vi "test FPGA.vi"() -> ()   [LabVIEW 2017]
uses:
  <vilib>/LabVIEW Targets/FPGA/cRIO/shared/nicrio_ModuleControls/nicrio_cRIO-9775_TriggerSlope.ctl
  <vilib>/LabVIEW Targets/FPGA/cRIO/shared/nicrio_ModuleControls/nicrio_BasicConversionTime.ctl
  <vilib>/LabVIEW Targets/FPGA/cRIO/shared/nicrio_ModuleControls/nicrio_cRIO-9775_RecordDataRates4ChansRing.ctl
  <vilib>/rvi/Emulation/niFpgaGetClockAttributes.vi
  <vilib>/rvi/Emulation/niFpgaSctlEmulationGetInTimedLoop.vi
  <vilib>/rvi/Emulation/niFpgaEmulationReportErrorSimple.vi
  <vilib>/rvi/eio/common/nirviEmuTemplateMethod_errors.vi
  <vilib>/rvi/Emulation/niFpgaCriticalErrorInLSC.vi
  <vilib>/rvi/eio/common/nirviEmuTemplatePropertySet_errors.vi
  <vilib>/rvi/interface/RandomDataEmulation/niFpgaRandomDataHandleErrors.vi
  <vilib>/eio/EIOMethodNode/EIOMethodNode.xnode
  <vilib>/eio/EIONode/EIONode.xnode
  <vilib>/eio/EIOPropertyNode/EIOPropertyNode.xnode
  <vilib>/rvi/DataTransferAndStorage/Container/XNode/niFpgaContainer.xnode
  <vilib>/rvi/interface/RandomDataEmulation/nirviRandomDataFpgaReadWriteTemplate.vi
  <vilib>/rvi/eio/common/nirviEmuTemplatePropertyGet_errors.vi
  <vilib>/rvi/eio/common/nirviEmuTemplatePropertyGet_noerrors.vi
  <vilib>/rvi/eio/common/nirviEmuTemplatePropertySet_noerrors.vi
panel:
  in  "stop":bool
  in  "Timeout":i32
  in  "Record Samples":u32=25
  in  "Record PreTrigger Samples":u32=1
  in  "Record Data Rate":T1=1 items=["20.000 MS/s (NI 9775)"=1, "10.00 MS/s (NI 9775)"=2, "6.667 MS/s (NI 9775)"=3, "5.000 MS/s (NI 9775)"=4, "2.500 MS/s (NI 9775)"=8, "1.667 MS/s (NI 9775)"=12, "1.250 MS/s (NI 9775)"=16, "1.000 MS/s (NI 9775)"=20, "833.333 KS/s (NI 9775)"=24, "714.286 KS/s (NI 9775)"=28, "625.000 KS/s (NI 9775)"=32, "555.556 KS/s (NI 9775)"=36, "500.000 KS/s (NI 9775)"=40, "454.545 KS/s (NI 9775)"=44, "416.667 KS/s (NI 9775)"=48, "384.615 KS/s (NI 9775)"=52, "357.143 KS/s (NI 9775)"=56, "333.333 KS/s (NI 9775)"=60, "312.500 KS/s (NI 9775)"=64, "294.118 KS/s (NI 9775)"=68, "277.778 KS/s (NI 9775)"=72, "263.158 KS/s (NI 9775)"=76, "250.000 KS/s (NI 9775)"=80, "238.095 KS/s (NI 9775)"=84, "227.273 KS/s (NI 9775)"=88, "217.391 KS/s (NI 9775)"=92, "208.333 KS/s (NI 9775)"=96, "200.000 KS/s (NI 9775)"=100, "192.308 KS/s (NI 9775)"=104, "185.185 KS/s (NI 9775)"=108, "178.571 KS/s (NI 9775)"=112, "172.414 KS/s (NI 9775)"=116, "166.667 KS/s (NI 9775)"=120, "161.290 KS/s (NI 9775)"=124, "156.250 KS/s (NI 9775)"=128, "151.515 KS/s (NI 9775)"=132, "147.059 KS/s (NI 9775)"=136, "142.857 KS/s (NI 9775)"=140, "138.889 KS/s (NI 9775)"=144, "135.135 KS/s (NI 9775)"=148, "131.579 KS/s (NI 9775)"=152, "128.205 KS/s (NI 9775)"=156, "125.000 KS/s (NI 9775)"=160, "121.951 KS/s (NI 9775)"=164, "119.048 KS/s (NI 9775)"=168, "116.279 KS/s (NI 9775)"=172, "113.636 KS/s (NI 9775)"=176, "111.111 KS/s (NI 9775)"=180, "108.696 KS/s (NI 9775)"=184, "106.383 KS/s (NI 9775)"=188, "104.167 KS/s (NI 9775)"=192, "102.041 KS/s (NI 9775)"=196, "100.000 KS/s (NI 9775)"=200, "50.000 KS/s (NI 9775)"=400, "33.333 KS/s (NI 9775)"=600, "25.000 KS/s (NI 9775)"=800, "20.000 KS/s (NI 9775)"=1000, "16.667 KS/s (NI 9775)"=1200, "14.286 KS/s (NI 9775)"=1400, "12.500 KS/s (NI 9775)"=1600, "11.111 KS/s (NI 9775)"=1800, "10.000 KS/s (NI 9775)"=2000, "9.091 KS/s (NI 9775)"=2200, "8.333 KS/s (NI 9775)"=2400, "7.692 KS/s (NI 9775)"=2600, "7.143 KS/s (NI 9775)"=2800, "6.667 KS/s (NI 9775)"=3000, "6.250 KS/s (NI 9775)"=3200, "5.882 KS/s (NI 9775)"=3400, "5.556 KS/s (NI 9775)"=3600, "5.000 KS/s (NI 9775)"=4000, "4.762 KS/s (NI 9775)"=4200, "4.545 KS/s (NI 9775)"=4400, "4.348 KS/s (NI 9775)"=4600, "4.167 KS/s (NI 9775)"=4800, "4.000 KS/s (NI 9775)"=5000, "3.846 KS/s (NI 9775)"=5200, "3.571 KS/s (NI 9775)"=5600, "3.333 KS/s (NI 9775)"=6000, "3.125 KS/s (NI 9775)"=6400, "2.941 KS/s (NI 9775)"=6800, "2.778 KS/s (NI 9775)"=7200, "2.632 KS/s (NI 9775)"=7600, "2.500 KS/s (NI 9775)"=8000, "2.381 KS/s (NI 9775)"=8400, "2.273 KS/s (NI 9775)"=8800, "2.174 KS/s (NI 9775)"=9200, "2.083 KS/s (NI 9775)"=9600, "2.000 KS/s (NI 9775)"=10000, "1.923 KS/s (NI 9775)"=10400, "1.852 KS/s (NI 9775)"=10800, "1.786 KS/s (NI 9775)"=11200, "1.724 KS/s (NI 9775)"=11600, "1.667 KS/s (NI 9775)"=12000, "1.613 KS/s (NI 9775)"=12400, "1.563 KS/s (NI 9775)"=12800, "1.515 KS/s (NI 9775)"=13200, "1.471 KS/s (NI 9775)"=13600, "1.429 KS/s (NI 9775)"=14000, "1.389 KS/s (NI 9775)"=14400, "1.351 KS/s (NI 9775)"=14800, "1.316 KS/s (NI 9775)"=15200, "1.282 KS/s (NI 9775)"=15600, "1.250 KS/s (NI 9775)"=16000, "1.220 KS/s (NI 9775)"=16400, "1.190 KS/s (NI 9775)"=16800, "1.163 KS/s (NI 9775)"=17200, "1.136 KS/s (NI 9775)"=17600, "1.111 KS/s (NI 9775)"=18000, "1.087 KS/s (NI 9775)"=18400, "1.064 KS/s (NI 9775)"=18800, "1.042 KS/s (NI 9775)"=19200, "1.020 KS/s (NI 9775)"=19600, "1.000 KS/s (NI 9775)"=20000, "0.980 KS/s (NI 9775)"=20400, "0.962 KS/s (NI 9775)"=20800, "0.943 KS/s (NI 9775)"=21200, "0.926 KS/s (NI 9775)"=21600, "0.909 KS/s (NI 9775)"=22000, "0.893 KS/s (NI 9775)"=22400, "0.877 KS/s (NI 9775)"=22800, "0.862 KS/s (NI 9775)"=23200, "0.847 KS/s (NI 9775)"=23600, "0.833 KS/s (NI 9775)"=24000, "0.820 KS/s (NI 9775)"=24400, "0.806 KS/s (NI 9775)"=24800, "0.794 KS/s (NI 9775)"=25200, "0.781 KS/s (NI 9775)"=25600, "0.694 KS/s (NI 9775)"=28800, "0.625 KS/s (NI 9775)"=32000, "0.568 KS/s (NI 9775)"=35200, "0.521 KS/s (NI 9775)"=38400, "0.446 KS/s (NI 9775)"=44800, "0.391 KS/s (NI 9775)"=51200, "0.347 KS/s (NI 9775)"=57600, "0.313 KS/s (NI 9775)"=64000]
  in  "Timing Mode":T2
  out "error out 3":errorcluster
  out "error out 2":errorcluster
  out "AI1":fxp<+/-,17,5>=0.1259765625
  in  "Points":i32=1
  in  "AI Trigger Configuration":T4={"Trigger Slope"=enum."Positive", "Trigger Level"=0.10009765625, "Hystesis Value"=0.090087890625, "AI Channel"=0}
  out "error out":errorcluster
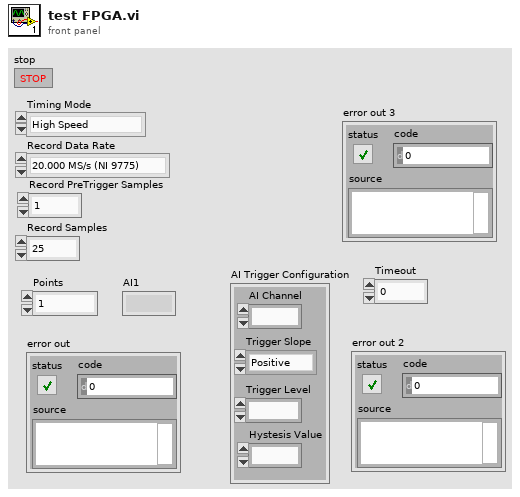
[diagram p1: front panel]
types:
  T1 = typedef "nicrio_cRIO-9775_RecordDataRates4ChansRing.ctl" = u16
  T2 = typedef "nicrio_BasicConversionTime.ctl" = enum8{"High Speed", "High Resolution"}
  T3 = typedef "nicrio_cRIO-9775_TriggerSlope.ctl" = enum8{"Positive", "Negative"}
  T4 = cluster{"Trigger Slope":T3, "Trigger Level":fxp<+/-,17,5>, "Hystesis Value":fxp<+,16,4>, "AI Channel":u8}
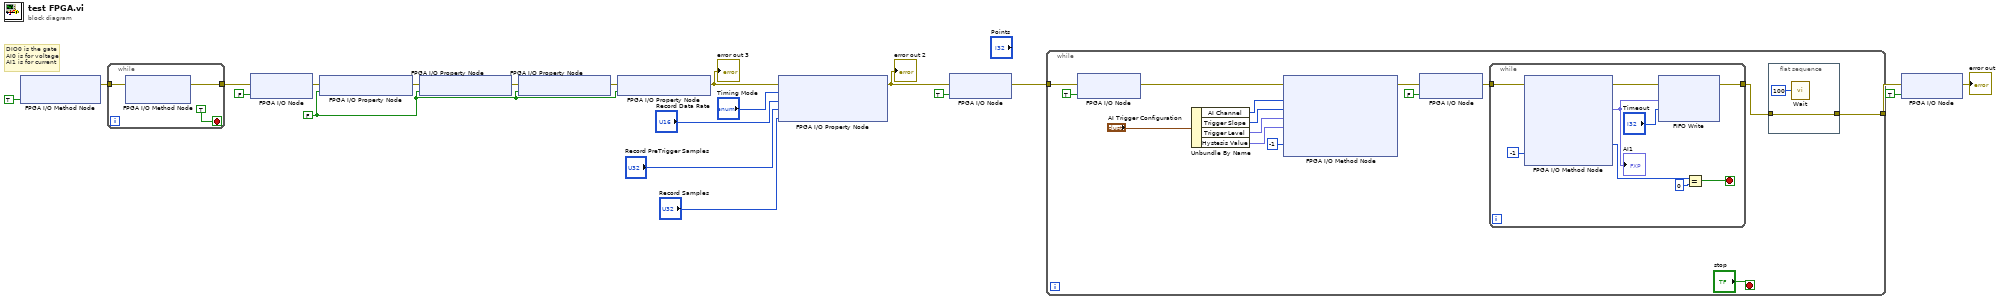
[diagram p0: block diagram]
diagram:
  w8 = FALSE ("Enable Low Pass Filter")
  # "DIO0 is the gate\nAI0 is for voltage\nAI1 is for current"
  n1 = xnode "FPGA I/O Method Node"("Enable"=TRUE) -> ("error out"=w16:errorcluster)  [unwired: 2 in, 1 out]
  n2 = while {
    tunnel: w16 -> [w23]
    tunnel: [w22] -> w15
    stop <- TRUE stop-if-true
    n3 = xnode "FPGA I/O Method Node"("error in"=w23) -> ("error out"=w22:errorcluster)  [unwired: 1 in, 2 out]
  }
  n4 = xnode "FPGA I/O Node"("error in"=w15, "Mod2/DIO0"=FALSE) -> ("error out"=w14:errorcluster)  [unwired: 1 in, 1 out]
  n5 = xnode "FPGA I/O Property Node"("error in"=w14, "Enable Low Pass Filter"=w8) -> ("error out"=w13:errorcluster)  [unwired: 1 in, 1 out]
  n6 = xnode "FPGA I/O Property Node"("error in"=w13, "Enable Low Pass Filter"=w8) -> ("error out"=w10:errorcluster)  [unwired: 1 in, 1 out]
  n7 = xnode "FPGA I/O Property Node"("error in"=w10, "Enable Low Pass Filter"=w8) -> ("error out"=w9:errorcluster)  [unwired: 1 in, 1 out]
  n8 = xnode "FPGA I/O Property Node"("error in"=w9, "Enable Low Pass Filter"=w8) -> ("error out"=w7:errorcluster)  [unwired: 1 in, 1 out]
  "error out 3" <- w7
  n9 = xnode "FPGA I/O Property Node"("error in"=w7, "Timing Mode"="Timing Mode", "Record Data Rate"="Record Data Rate", "Record PreTrigger Samples"="Record PreTrigger Samples", "Record Samples"="Record Samples") -> ("error out"=w6:errorcluster)  [unwired: 1 in, 1 out]
  "error out 2" <- w6
  n10 = xnode "FPGA I/O Node"("error in"=w6, "Mod1/Start"=TRUE) -> ("error out"=w12:errorcluster)  [unwired: 1 in, 1 out]
  n11 = while {
    tunnel: w12 -> [w38]
    tunnel: [w24] -> w1
    stop <- "stop" stop-if-true
    n12 = xnode "FPGA I/O Node"("error in"=w38, "Mod2/DIO0"=TRUE) -> ("error out"=w31:errorcluster)  [unwired: 1 in, 1 out]
    n13 = Unbundle By Name("AI Trigger Configuration") -> ("AI Channel"=w35:u8, "Trigger Slope"=w34:T3, "Trigger Level"=w33:fxp<+/-,17,5>, "Hystesis Value"=w32:fxp<+,16,4>)
    n14 = xnode "FPGA I/O Method Node"("error in"=w31, "AI Channel"=w35, "Trigger Slope"=w34, "Trigger Level"=w33, "Hysteresis Value"=w32, "Timeout (Ticks)"=-1) -> ("error out"=w29:errorcluster)  [unwired: 1 in, 3 out]
    n15 = xnode "FPGA I/O Node"("error in"=w29, "Mod2/DIO0"=FALSE) -> ("error out"=w28:errorcluster)  [unwired: 1 in, 1 out]
    n16 = while {
      tunnel: w28 -> [w49]
      tunnel: [w41] -> w25
      stop <- w45 stop-if-true
      n17 = xnode "FPGA I/O Method Node"("error in"=w49, "Timeout (Ticks)"=-1) -> ("error out"=w43:errorcluster, "AI1"=w42:fxp<+/-,17,5>, "Elements Remaining"=w47:u32)  [unwired: 1 in, 6 out]
      "AI1" <- w42
      n18 = xnode ("FIFO Write")("Element"=w42, "Timeout"="Timeout", "error in (no error)"=w43) -> ("error out"=w41:errorcluster)  [unwired: 1 in, 2 out]
      n19 = Equal?(x=w47, y=u32 0) -> (x = y?=w45:bool)
    }
    n20 = flat-sequence {
      tunnel: w25 -> [w40]
      tunnel: [w40] -> w24
      frame #0 {
        n21 = call "Wait"("Count(uSec)"=u32 100) -> ()  [unwired: 1 out]
      }
    }
  }
  n22 = xnode "FPGA I/O Node"("error in"=w1, "Mod1/Stop"=TRUE) -> ("error out"=→"error out":errorcluster)  [unwired: 1 in, 1 out]
